vi "Motic Set Trigger Type.vi"(8 "error in (no error)":errorcluster, 10 "trigger type":u32(ring) items=["Free", "Software", "Hardware-Rise", "Hardware-Fall"], 11 "camera":i32) -> (0 "error out":errorcluster, 3 "camera out":i32)   [LabVIEW 2012, in "MoticApi.lvlib"]
doc: "MOTICAPI bool Motic_SetTriggerType(MUCam_Handle camera, MUCam_Trigger_Type type);"
uses:
  MoticApi.lvlib
  MoticApi.dll
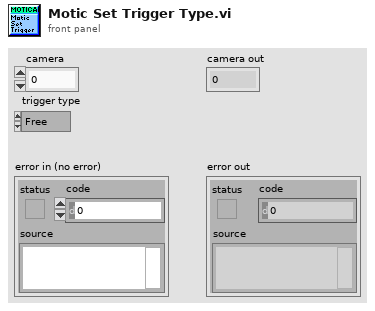
[diagram p1: front panel]
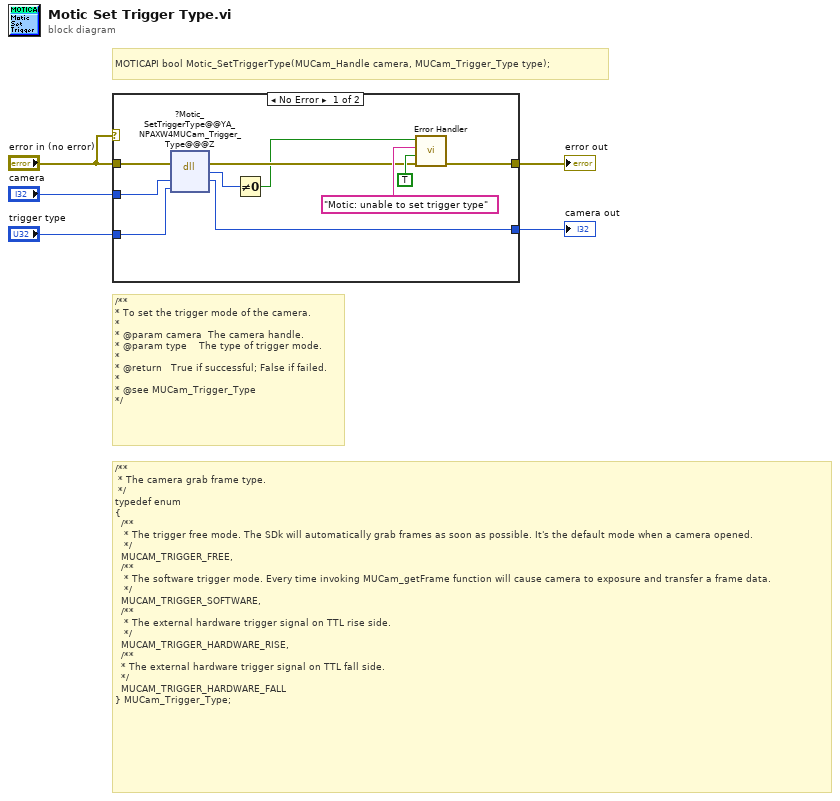
[diagram p0: block diagram]
diagram:
  # "/**\n * The camera grab frame type.\n */\ntypedef enum\n{\n  /**\n   * The trigger free mode. The SDk will automatically grab frames as soon as possible. It's the default mode when a camera opened.\n   */\n  MUCAM_TRIGGER_FREE,\n  /**\n   * The software trigger mode. Every time invoking MUCam_getFrame function will cause camera to exposure and transfer a frame data.\n   */\n  MUCAM_TRIGGER_SOFTWARE,\n  /**\n   * The external hardware trigger signal on TTL rise side.\n   */\n  MUCAM_TRIGGER_HARDWARE_RISE,\n  /**\n  * The external hardware trigger signal on TTL fall side.\n  */\n  MUCAM_TRIGGER_HARDWARE_FALL\n} MUCam_Trigger_Type;"
  # "/**\n* To set the trigger mode of the camera.\n*\n* @param camera  The camera handle.\n* @param type    The type of trigger mode.\n*\n* @return   True if successful; False if failed.\n*\n* @see MUCam_Trigger_Type\n*/"
  # "MOTICAPI bool Motic_SetTriggerType(MUCam_Handle camera, MUCam_Trigger_Type type);"
  n1 = case shown="No Error" "error in (no error)" {
    tunnel: "camera" -> [w14 w16]
    tunnel: [w13 w16] -> w4
    tunnel: "trigger type" -> [w12 _]
    tunnel: [w9 w17] -> w2
    tunnel: "error in (no error)" -> [w7 w17]
    frame No Error {
      n2 = dll-call lib="C:/Users/TTS-Digital/Desktop/MoticApi/MoticApi_git/MoticApi/MoticApi.*" fn="?Motic_SetTriggerType@@YA_NPAXW4MUCam_Trigger_Type@@@Z"(error in=w7, "camera"=w14, "type"=w12) -> (error out=w8:errorcluster, "return type"=w15:u8, "camera"=w13:i32)  [unwired: 3 in, 1 out]
      n3 = Not Equal To 0?(x=w15) -> (x != 0?=w6:bool)
      n4 = call "Error Handler.vi"("error in (no error)"=w8, "Is warning?"=TRUE, "Error message"="Motic: unable to set trigger type", "Function return"=w6) -> ("error out"=w9:errorcluster)  [unwired: 7 in]
    }
    frame Error {
    }
  }
  "camera out" <- w4
  "error out" <- w2
